vi "Pockels Cal_Error reporting.vi"(8 "error in (no error)":errorcluster, 10 "error IO":errorcluster, 11 "Function":T1) -> (0 "error out":errorcluster)   [LabVIEW 2020]
uses:
  Typedefs/Functional global standard states.ctl
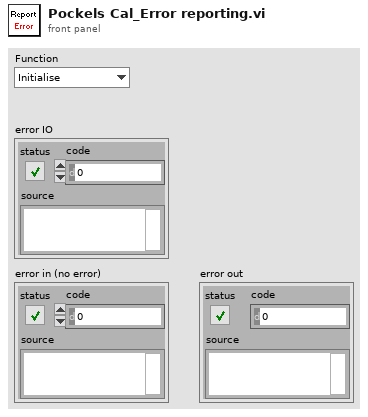
[diagram p1: front panel]
types:
  T1 = typedef "Functional global standard states.ctl" = enum16{"Initialise", "Read", "Write", "Load", "Save", "Clear"}
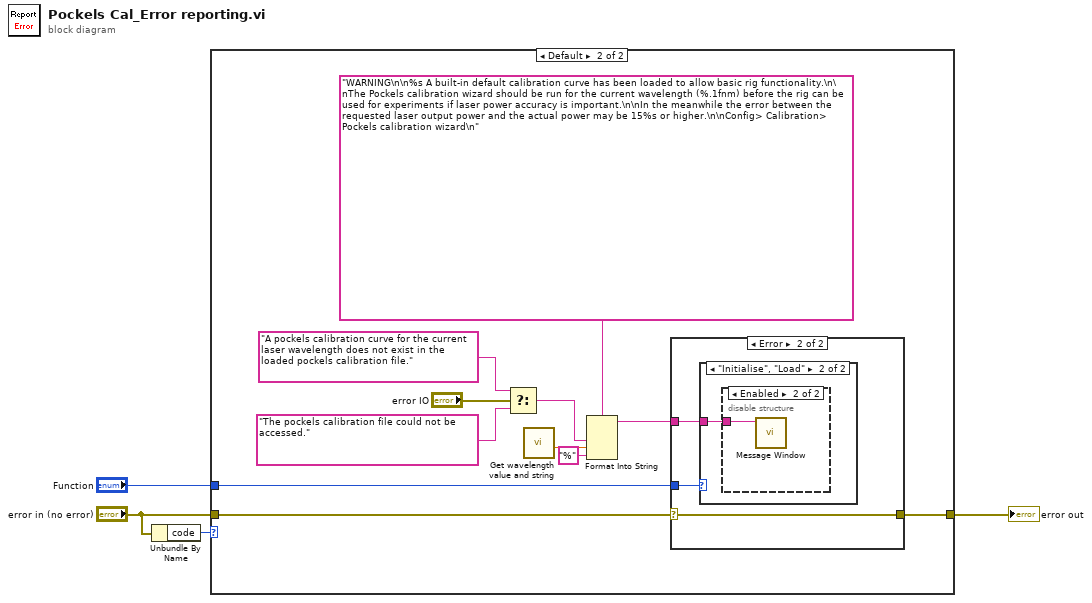
[diagram p0: block diagram]
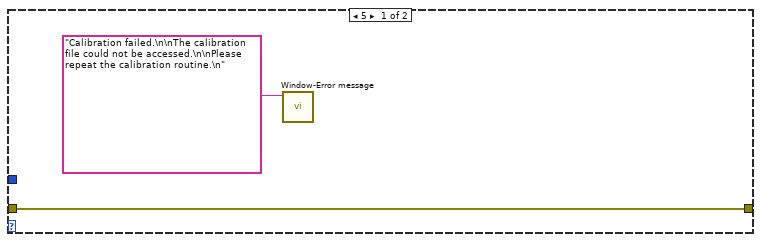
[diagram p2: hidden frame]
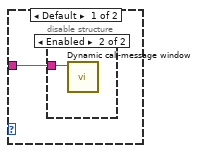
[diagram p4: hidden frame]
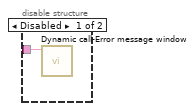
[diagram p5: hidden frame]
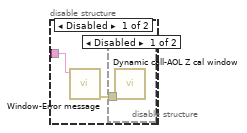
[diagram p6: hidden frame]
diagram:
  n1 = Unbundle By Name("error in (no error)") -> ("code"=w1:i32)
  n2 = case shown="Default" w1 {
    tunnel: [w5 w12] -> w4
    tunnel: "error in (no error)" -> [w5 w11]
    tunnel: "Function" -> [_ w10]
    frame 5 {
      n3 = call "Window-Error message.vi"("Message"="Calibration failed.\n\nThe calibration file could not be accessed.\n\nPlease repeat the calibration routine.\n") -> ()  [unwired: 10 in, 1 out]
    }
    frame Default {
      n4 = Select(t="A pockels calibration curve for the current laser wavelength does not exist in the loaded pockels calibration file." ("Error Message"), s="error IO", f="The pockels calibration file could not be accessed." ("Error Message")) -> (s? t:f=w17:string)
      n5 = call "Get wavelength value and string.vi"() -> ("Wavelength value"=w8:dbl)  [unwired: 9 in, 2 out]
      n6 = Format Into String(format string="WARNING\n\n%s A built-in default calibration curve has been loaded to allow basic rig functionality.\n\nThe Pockels calibration wizard should be run for the current wavelength (%.1fnm) before the rig can be used for experiments if laser power accuracy is important.\n\nIn the meanwhile the error between the requested laser output power and the actual power may be 15%s or higher.\n\nConfig> Calibration> Pockels calibration wizard\n" ("Error Message"), w17, w8, "%" ("input 3")) -> (resulting string=w14:string)  [unwired: 2 in, 1 out]
      n7 = case shown="Error" w11 {
        selector: w11 -> [w18 w21]
        tunnel: [w18 w21] -> w12
        tunnel: w14 -> [_ w19]
        tunnel: w10 -> [_ w20]
        frame No Error {
        }
        frame Error {
          n8 = case shown="\"Initialise\", \"Load\"" w20 {
            tunnel: w19 -> [w22 w25]
            frame Default {
              n9 = disable-structure shown="Enabled" {
                disable-tunnel: w22 -> [w23 w24]
                frame Disabled {
                  n10 = call "Dynamic call-Error message window.vi"("Error Message"=w23) -> ()  [unwired: 10 in, 1 out]
                }
                frame Enabled {
                  n11 = call "Dynamic call-message window.vi"("Message"=w24) -> ()  [unwired: 10 in, 1 out]
                }
              }
            }
            frame "Initialise", "Load" {
              n12 = disable-structure shown="Enabled" {
                disable-tunnel: w25 -> [w27 w29]
                frame Disabled {
                  n13 = call "Window-Error message.vi"("Message"=w27) -> ("Error Out (no error)"=w26:errorcluster)  [unwired: 10 in]
                  n14 = disable-structure shown="Disabled" {
                    disable-tunnel: w26 -> [w28 _]
                    frame Disabled {
                      n15 = call "Dynamic call-AOL Z cal window.vi"("error in (no error)"=w28) -> ()  [unwired: 10 in, 1 out]
                    }
                    frame Enabled {
                    }
                  }
                }
                frame Enabled {
                  n16 = call "Message Window.vi"("Message string"=w29) -> ()  [unwired: 10 in, 1 out]
                }
              }
            }
          }
        }
      }
    }
  }
  "error out" <- w4
